vi "Swerve Wheel PercentVBus.vi"(10 "Input Array":dbl[](array[numeric]), 11 "Wheel":T1(ring)) -> ()   [LabVIEW 2016]
uses:
  <vilib>/Rock Robotics/Network Tables/NT Read Number.vi
  <vilib>/Rock Robotics/Network Tables/NT Write Number.vi
  <vilib>/addons/control/pid/pid.llb/PID (DBL).vi
  <vilib>/addons/control/pid/NI_PID_pid.lvlib
panel:
  in  "Deadband":dbl
  out "Drive Output":dbl
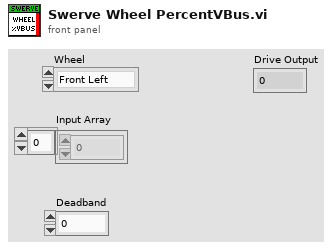
[diagram p1: front panel]
types:
  T1 = enum16{"Front Left", "Front Right", "Back Left", "Back Right"}
  T2 = cluster{"proportional gain (Kc)":dbl, "integral time (Ti, min)":dbl, "derivative time (Td, min)":dbl}
  T3 = enum16{"Z", "Y", "X", "Rot. Point X", "Rot. Point Y", "Width/2", "Max", "Length/2"}
  T4 = enum16{"Z Axis", "Y", "X", "Rot. Point X", "Rot. Point Y", "Width/2", "Max", "Length/2"}
  T5 = typedef "WPI_MotorControlDeviceRef.ctl" = cluster{"DeviceStatus":errorcluster, "Type":T6, "PWM":cluster{"PWM Channel":T7, "DeadBand":T8}, "CAN":cluster{"Device Number":u8, "SetOutput VI Ref":variant, "GetOutput VI Ref":variant, "Enable VI Ref":variant, "Disable VI Ref":variant, "Data":variant}, "Invert":bool}
  T6 = typedef "WPI_MotorControlType.ctl" = enum16{"PWM", "CAN"}
  T7 = typedef "FPGA_DIOPWMChannel.ctl" = enum8{"PWM 0", "PWM 1", "PWM 2", "PWM 3", "PWM 4", "PWM 5", "PWM 6", "PWM 7", "PWM 8", "PWM 9", "PWM MXP 0", "PWM MXP 1", "PWM MXP 2", "PWM MXP 3", "PWM MXP 4", "PWM MXP 5", "PWM MXP 6", "PWM MXP 7", "PWM MXP 8", "PWM MXP 9", "Invalid"}
  T8 = typedef "WPI_PWMDeadband.ctl" = cluster{"Name":string, "maxPositivePwm":i32, "minPositivePwm":i32, "centerPwm":i32, "maxNegativePwm":i32, "minNegativePwm":i32, "angularRange":u16}
  T9 = typedef "WPI_CANTalonSRX_GlobalStatus.ctl" = cluster{"Applied Throttle":dbl, "Module Enabled":bool, "CAN Error":errorcluster, "Closed Loop Error":dbl, "Forward Limit Switch Closed":bool, "Reverse Limit Switch Closed":bool, "Sensor Position":dbl, "Sensor Velocity":dbl, "Current":dbl, "Sticky Fault - Over Temp":bool, "Sticky Fault - Under Voltage":bool, "Sticky Fault - Forward Limit":bool, "Sticky Fault - Reverse Limit":bool, "Sticky Fault - Forward Soft Limit":bool, "Sticky Fault - Reverse Soft Limit":bool, "Brake is Enabled":bool, "Encoder Position":dbl, "Encoder Velocity":dbl, "Encoder Index Count":dbl, "Encoder A Pin State":bool, "Encoder B Pin State":bool, "Encoder Index Pin State":bool, "Analog In":dbl, "Analog In Velocity":dbl, "Temperature (C)":dbl, "Battery Voltage":dbl, "Control 5 Is Supported":bool, "Current Profile Slot Select":dbl, "Pos Div 8":bool, "Vel Div 4":bool, "Pulse Width Position":i32, "Pulse Width Velocity":i32, "Pulse Width Rise To Rise (us)":i32, "Pulse Width Rise To Fall (us)":i32, "Mot Prof Active Is Under Run":bool, "Mot Prof Active Has Under Run":bool, "Mot Prof Active Is Last":bool, "Mot Prof Active Velocity Only":bool, "Mot Prof Active Is Valid":bool, "Mot Prof Buffer Is Full":bool, "Mot Prof Active Profile Slot Select":i32, "Mot Prof NextID":i32, "Mot Prof Count":i32, "Mot Prof Active Velocity":dbl, "Mot Prof Active Position":dbl, "Mot Prof Output Enable":i32, "UsageFrame":u32}
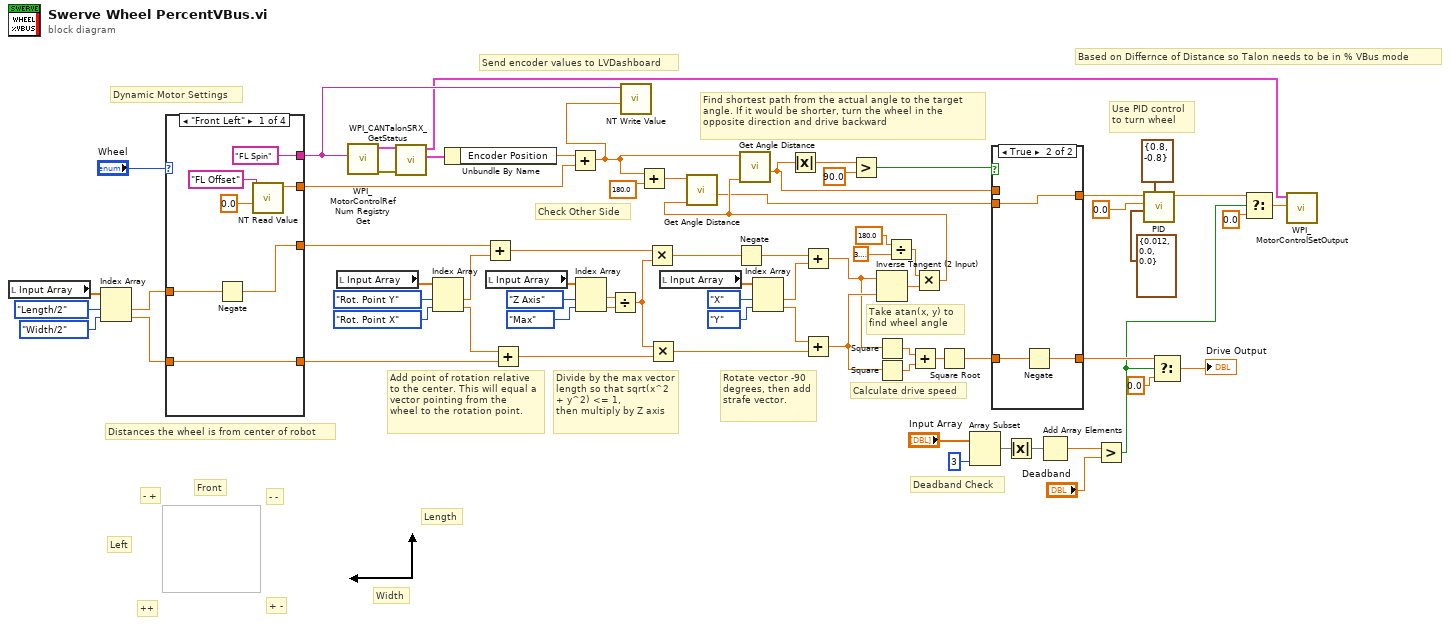
[diagram p0: block diagram]
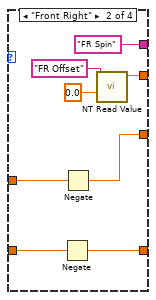
[diagram p3: hidden frame]
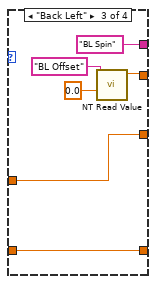
[diagram p4: hidden frame]
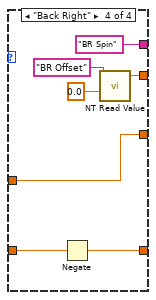
[diagram p5: hidden frame]
diagram:
  # "Based on Differnce of Distance so Talon needs to be in % VBus mode"
  # "Use PID control\nto turn wheel"
  # "Check Other Side"
  # "Take atan(x, y) to find wheel angle"
  # "Calculate drive speed"
  # "- -"
  # "+ -"
  # "++"
  # "- +"
  # "Width"
  # "Length"
  # "Left"
  # "Front"
  # "Distances the wheel is from center of robot"
  # "Dynamic Motor Settings"
  # "Divide by the max vector length so that sqrt(x^2 + y^2) <= 1,\nthen multiply by Z axis"
  # "Add point of rotation relative to the center. This will equal a vector pointing from the\nwheel to the rotation point."
  # "Rotate vector -90 degrees, then add strafe vector."
  # "Deadband Check"
  # "Find shortest path from the actual angle to the target angle. If it would be shorter, turn the wheel in the opposite direction and drive backward"
  # "Send encoder values to LVDashboard"
  n1 = local read "Input Array"() -> (w36:dbl[])
  n2 = Index Array(array=w36, index #1=T3."Length/2", index #2=T3."Width/2") -> (element #1=w32:dbl, element #2=w31:dbl)
  n3 = case shown="\"Front Left\"" "Wheel" {
    tunnel: ["FL Spin" ("refnum name") "FR Spin" ("refnum name") "BL Spin" ("refnum name") "BR Spin" ("refnum name")] -> w68
    tunnel: [w76 w84 w90 w97] -> w1
    tunnel: [w73 w81 w89 w96] -> w34
    tunnel: w32 -> [w75 w83 w89 w96]
    tunnel: [w74 w80 w88 w94] -> w33
    tunnel: w31 -> [w74 w82 w88 w95]
    frame "Front Left" {
      n4 = Negate(x=w75) -> (-x=w73:dbl)
      n5 = call-poly <vilib>:"NT Read Value.vi"("Default Value"=0.0, "Name"="FL Offset") -> ("Numeric"=w76:dbl)  [unwired: 8 in, 1 out]
    }
    frame "Front Right" {
      n6 = Negate(x=w82) -> (-x=w80:dbl)
      n7 = Negate(x=w83) -> (-x=w81:dbl)
      n8 = call-poly <vilib>:"NT Read Value.vi"("Default Value"=0.0, "Name"="FR Offset") -> ("Numeric"=w84:dbl)  [unwired: 8 in, 1 out]
    }
    frame "Back Left" {
      n9 = call-poly <vilib>:"NT Read Value.vi"("Default Value"=0.0, "Name"="BL Offset") -> ("Numeric"=w90:dbl)  [unwired: 8 in, 1 out]
    }
    frame "Back Right" {
      n10 = Negate(x=w95) -> (-x=w94:dbl)
      n11 = call-poly <vilib>:"NT Read Value.vi"("Default Value"=0.0, "Name"="BR Offset") -> ("Numeric"=w97:dbl)  [unwired: 8 in, 1 out]
    }
  }
  n12 = local read "Input Array"() -> (w57:dbl[])
  n13 = call <vilib>:"WPI_MotorControlRefNum Registry Get.vi"("refnum name"=w68) -> ("error out"=w70:errorcluster, "MotorControlDevRef"=w71:T5)  [unwired: 9 in]
  n14 = call <vilib>:"WPI_CANTalonSRX_GetStatus.vi"("error in (no error)"=w70, "CAN Talon SRX Ref"=w71) -> ("Talon SRX Status"=w69:T9, "CAN Talon SRX Ref"=w6:T5)  [unwired: 7 in, 1 out]
  n15 = Index Array(array=w57, index #1=T3."Rot. Point Y", index #2=T3."Rot. Point X") -> (element #1=w54:dbl, element #2=w55:dbl)
  n16 = Unbundle By Name(w69) -> ("Encoder Position"=w67:dbl)
  n17 = Add(x=w34, y=w54) -> (x+y=w38:dbl)
  n18 = local read "Input Array"() -> (w52:dbl[])
  n19 = Add(x=w55, y=w33) -> (x+y=w48:dbl)
  n20 = Add(x=w67, y=w1) -> (x+y=w2:dbl)
  n21 = Index Array(array=w52, index #1=T4."Z Axis", index #2=T3."Max") -> (element #1=w49:dbl, element #2=w50:dbl)
  n22 = Divide(x=w49, y=w50) -> (x/y=w47:dbl)
  n23 = call-poly <vilib>:"NT Write Value.vi"("Numeric"=w2, "Name"=w68) -> ()  [unwired: 9 in, 1 out]
  n24 = Add(x=w2, y=180.0) -> (x+y=w18:dbl)
  n25 = Multiply(x=w38, y=w47) -> (x*y=w40:dbl)
  n26 = Multiply(x=w47, y=w48) -> (x*y=w43:dbl)
  n27 = local read "Input Array"() -> (w45:dbl[])
  n28 = Negate(x=w40) -> (-x=w39:dbl)
  n29 = Index Array(array=w45, index #1=T3."X", index #2=T3."Y") -> (element #1=w41:dbl, element #2=w42:dbl)
  n30 = Add(x=w39, y=w41) -> (x+y=w22:dbl)
  n31 = Add(x=w42, y=w43) -> (x+y=w23:dbl)
  n32 = Inverse Tangent (2 Input)(1:w23, 2:w22) -> (0:w30:dbl)
  n33 = Square(x=w22) -> (x^2=w24:dbl)
  n34 = Square(x=w23) -> (x^2=w29:dbl)
  n35 = Divide(x=180.0 ("y"), y=3.141592653589793) -> (x/y=w27:dbl)
  n36 = Add(x=w24, y=w29) -> (x+y=w28:dbl)
  n37 = Multiply(x=w27, y=w30) -> (x*y=w21:dbl)
  n38 = call "Get Angle Distance.vi"("Target"=w21, "Current"=w18) -> ("Distance"=w15:dbl)  [unwired: 9 in]
  n39 = call "Get Angle Distance.vi"("Target"=w21, "Current"=w2) -> ("Distance"=w14:dbl)  [unwired: 9 in]
  n40 = Absolute Value(x=w14) -> (abs(x)=w19:dbl)
  n41 = Greater?(x=w19, y=90.0) -> (0:w16:bool)
  n42 = Square Root(x=w28) -> (sqrt(x)=w12:dbl)
  n43 = Array Subset(array="Input Array", length=3) -> (w64:dbl[])  [unwired: 1 in]
  n44 = case shown="True" w16 {
    tunnel: w15 -> [_ w103]
    tunnel: w14 -> [w102 _]
    tunnel: [w101 w104] -> w13
    tunnel: w12 -> [w101 w105]
    tunnel: [w102 w103] -> w5
    frame False {
    }
    frame True {
      n45 = Negate(x=w105) -> (-x=w104:dbl)
    }
  }
  n46 = Absolute Value(x=w64) -> (abs(x)=w62:dbl[])
  n47 = Add Array Elements(numeric array=w62) -> (sum=w60:dbl)
  n48 = Greater?(x=w60, y="Deadband") -> (0:w4:bool)
  n49 = call-poly <vilib>:"PID.vi"("output range"=cluster{"output high":dbl, "output low":dbl} {"output high"=0.8, "output low"=-0.8}, "PID gains"=T2 {"proportional gain (Kc)"=0.012, "integral time (Ti, min)"=0.0, "derivative time (Td, min)"=0.0}, "process variable"=0.0, "setpoint"=w5) -> ("output"=w7:dbl)  [unwired: 6 in, 1 out]
  n50 = Select(t=w13, s=w4, f=0.0) -> (s? t:f=→"Drive Output":dbl)
  n51 = Select(t=w7, s=w4, f=0.0) -> (s? t:f=w9:dbl)
  n52 = call <vilib>:"WPI_MotorControlSetOutput.vi"("Output"=w9, "MotorControlDevRef"=w6) -> ()  [unwired: 7 in, 3 out]
